vi "获取简易流程名称.vi"(0 "参数下拉列表":u16) -> (14 "字符串与值[]":T1)   [LabVIEW 2016, in "斯坦道氨氮.lvlib"]
uses:
  <vilib>/Utility/miscctls.llb/LVStringsAndValuesArrayTypeDef_U16.ctl
panel:
  in  "简易流程":u16(ring) items=["注射泵/多通阀复位"=0, "试剂填充"=1, "纯水填充"=2, "水样填充"=3, "标样核查标液填充"=4, "零点核查标液填充"=6, "跨度核查标液填充"=7, "消解池清洗"=11, "注射泵/储液环清洗"=12, "LED灯值测试"=13, "高温高压阀测试"=18, "消解加热测试"=19, "管路清洗排空"=24, "其他流程1"=30, "其他流程2"=31, "其他流程3"=32]
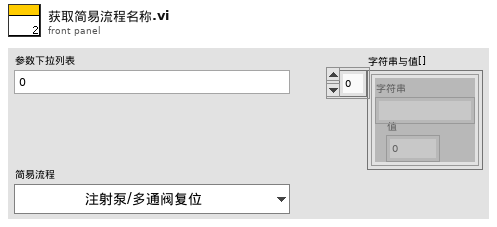
[diagram p1: front panel]
types:
  T1 = typedef "LVStringsAndValuesArrayTypeDef_U16.ctl" = cluster{"String":string, "Value":u16}[]
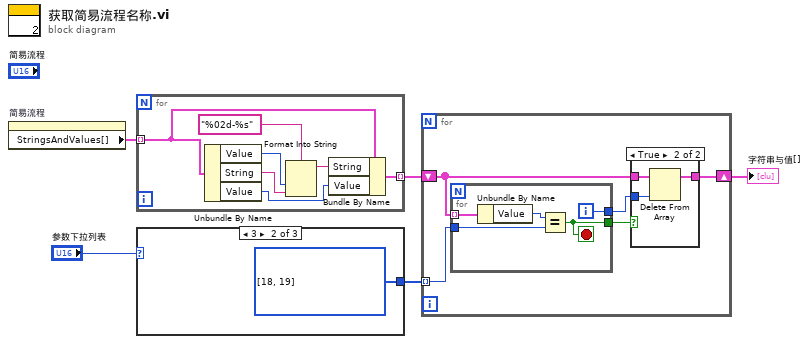
[diagram p0: block diagram]
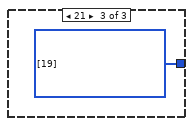
[diagram p3: hidden frame]
diagram:
  n1 = property on="简易流程" class="Ring (strict)"() -> ("StringsAndValues[]"=w2:T1)  [unwired: 2 in, 2 out]
  n2 = for {
    tunnel: w2 -> [w9] mode=indexing
    tunnel: [w7] -> w1 mode=indexing
    n3 = Unbundle By Name(w9) -> ("Value"=w11:u16, "String"=w10:string, "Value"=w6:u16)
    n4 = Format Into String(format string="%02d-%s" ("格式字符串"), w11, w10) -> (resulting string=w8:string)  [unwired: 2 in, 1 out]
    n5 = Bundle By Name(cluster=w9, "String"=w8, "Value"=w6) -> (w7:cluster{"String":string, "Value":u16})
  }
  n6 = case shown="3" "参数下拉列表" {
    tunnel: [_ u16[] [18, 19] ("索引") u16[] [19] ("索引")] -> w4
    frame 0, Default {
    }
    frame 3 {
    }
    frame 21 {
    }
  }
  n7 = for {
    shift-right: [w19] -> w3
    shift-left: w1 -> [w18]
    tunnel: w4 -> [w17] mode=indexing
    n8 = for {
      tunnel: w18 -> [w28] mode=indexing
      tunnel: w17 -> [w27]
      tunnel: [w24] -> w16
      tunnel: [w25] -> w15
      i -> [w24]
      stop <- w25 stop-if-true
      n9 = Unbundle By Name(w28) -> ("Value"=w26:u16)
      n10 = Equal?(x=w26, y=w27) -> (x = y?=w25:bool)
    }
    n11 = case shown="True" w15 {
      tunnel: [w20 w23] -> w19
      tunnel: w18 -> [w20 w22]
      tunnel: w16 -> [_ w21]
      frame False {
      }
      frame True {
        n12 = Delete From Array(array=w22, index=w21) -> (array with subset deleted=w23:cluster{"String":string, "Value":u16}[])  [unwired: 1 in, 1 out]
      }
    }
  }
  "字符串与值[]" <- w3
